vi "Read Access Token.vi"(8 "error in":errorcluster, 10 "password":string, 11 "username":string) -> (0 "error out":errorcluster, 2 "token":string)   [LabVIEW 2013, in "Particle API.lvlib"]
uses:
  Particle API.lvlib
  <vilib>/Utility/error.llb/Error Cluster From Error Code.vi
  <vilib>/ErrorRing/Error Ring.xnode
  <vilib>/httpClient/LabVIEWHTTPClient.lvlib
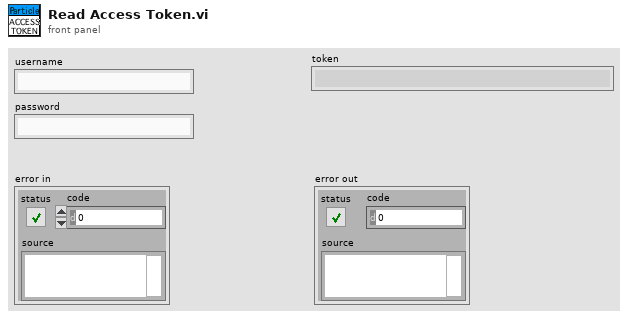
[diagram p1: front panel]
types:
  T1 = cluster{"token":string, "expires_at":string, "client":string}[]
  T2 = typedef "LabVIEWHTTPClient.lvlib/ClientHandle.ctl" = refnum<k1>
  T3 = typedef "Particle API.lvlib/Token Response JSON.ctl" = cluster{"access_token":string, "token_type":string, "expires_in":dbl, "refresh_token":string}
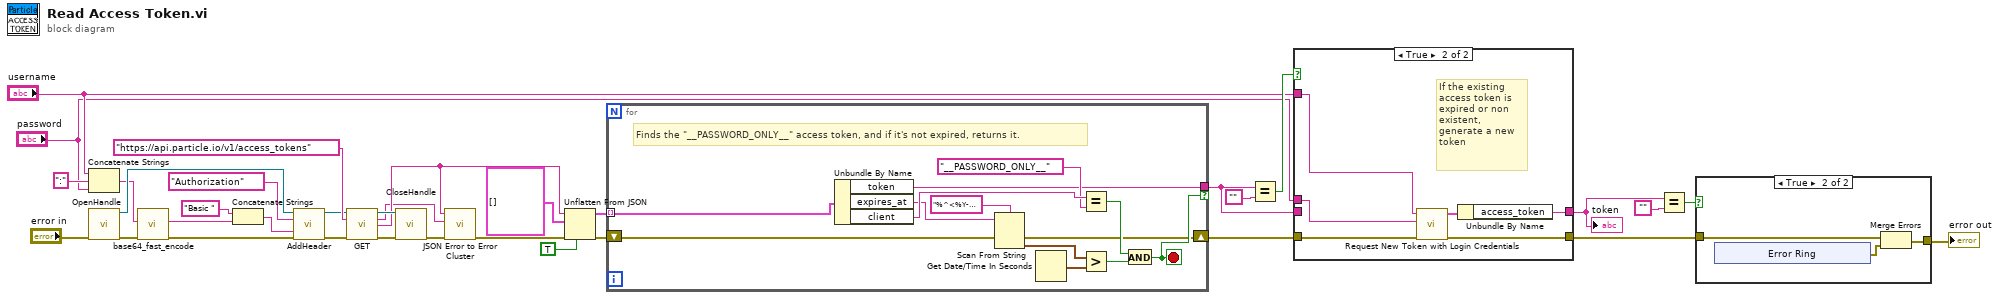
[diagram p0: block diagram]
diagram:
  n1 = Concatenate Strings("username", ":" ("string"), "password") -> (w24:string)
  n2 = call <vilib>:"OpenHandle.vi"("error in (no error)"="error in") -> ("client handle out"=w31:T2, "error out"=w27:errorcluster)  [unwired: 13 in]
  n3 = call "base64_fast_encode.vi"("error in (no error)"=w27, "string in (not encoded)"=w24) -> ("error out"=w28:errorcluster, "string out (base64-encoded)"=w22:string)  [unwired: 8 in]
  n4 = Concatenate Strings("Basic " ("string"), w22) -> (w23:string)
  n5 = call <vilib>:"AddHeader.vi"("client handle"=w31, "header"="Authorization", "value"=w23, "error in (no error)"=w28) -> ("client handle out"=w30:T2, "error out"=w32:errorcluster)  [unwired: 10 in]
  n6 = call <vilib>:"GET.vi"("client handle"=w30, "url"="https://api.particle.io/v1/access_tokens", "error in (no error)"=w32) -> ("client handle out"=w14:T2, "headers"=w10:string, "body"=w11:string, "error out"=w19:errorcluster)  [unwired: 9 in]
  n7 = call <vilib>:"CloseHandle.vi"("client handle"=w14, "error in (no error)"=w19) -> ("error out"=w13:errorcluster)  [unwired: 13 in]
  n8 = call "JSON Error to Error Cluster.vi"("error in (no error)"=w13, "headers"=w10, "JSON string"=w11) -> ("error out"=w12:errorcluster)  [unwired: 8 in]
  n9 = Unflatten From JSON(JSON string=w11, type and defaults=T1 [], default null elements? (F)=TRUE, error in (no error)=w12) -> (value=w20:T1, error out=w18:errorcluster)  [unwired: 3 in]
  n10 = for {
    tunnel: w20 -> [w47] mode=indexing
    tunnel: [w44] -> w5 if=w37
    shift-right: [w35] -> w8
    shift-left: w18 -> [w36]
    stop <- w37 stop-if-true
    # "Finds the \"__PASSWORD_ONLY__\" access token, and if it's not expired, returns it."
    n11 = Unbundle By Name(w47) -> ("token"=w44:string, "expires_at"=w42:string, "client"=w46:string)
    n12 = Scan From String(format string="%^<%Y-%m-%dT%H:%M:%S%3uZ>T", input string=w42, error in=w36) -> (error out=w35:errorcluster, output 1=w41:timestamp)  [unwired: 2 in, 2 out]
    n13 = Get Date/Time In Seconds() -> (seconds since 1Jan1904=w40:timestamp)
    n14 = Equal?(x=w46, y="__PASSWORD_ONLY__") -> (x = y?=w38:bool)
    n15 = Greater?(x=w41, y=w40) -> (0:w39:bool)
    n16 = And(x=w38, y=w39) -> (x .and. y?=w37:bool)
  }
  n17 = Equal?(x=w5, y="") -> (x = y?=w4:bool)
  n18 = case shown="True" w4 {
    tunnel: [w49 w50] -> w9
    tunnel: w5 -> [w49 _]
    tunnel: w8 -> [w48 w53]
    tunnel: [w48 w52] -> w7
    tunnel: "username" -> [_ w55]
    tunnel: "password" -> [_ w54]
    frame False {
    }
    frame True {
      # "If the existing access token is expired or non existent, generate a new token"
      n19 = call "Request New Token with Login Credentials.vi"("error in"=w53, "password"=w54, "username"=w55) -> ("error out"=w52:errorcluster, "token response"=w51:T3)  [unwired: 7 in]
      n20 = Unbundle By Name(w51) -> ("access_token"=w50:string)
    }
  }
  "token" <- w9
  n21 = Equal?(x=w9, y="") -> (x = y?=w15:bool)
  n22 = case shown="True" w15 {
    tunnel: w7 -> [w56 w58]
    tunnel: [w56 w57] -> w16
    frame False {
    }
    frame True {
      n23 = xnode "Error Ring"() -> ("error out"=w59:errorcluster)
      n24 = Merge Errors(w58, w59) -> (w57:errorcluster)
    }
  }
  "error out" <- w16
